vi "DistanciaRoboInimigoBola.vi"(7 "id inimigo":u32, 8 "Y bola":dbl format="%#_13g", 9 "X bola":dbl format="%#_13g", 10 "Y inimigo":dbl format="%#_13g", 11 "X inimigo":dbl format="%#_13g") -> (0 "id inimigo":u32, 3 "Distância":dbl format="%#_13g")   [LabVIEW 2017]
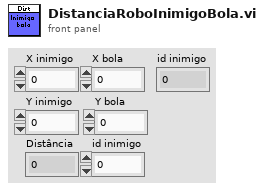
[diagram p1: front panel]
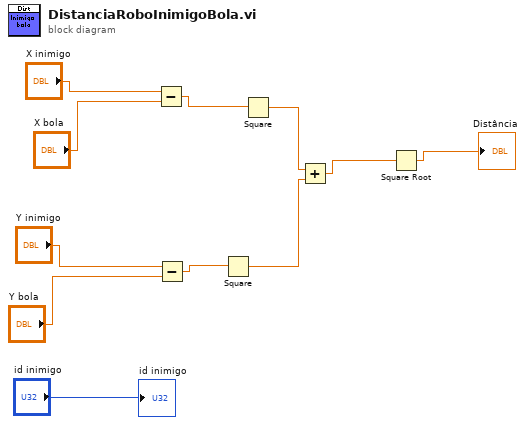
[diagram p0: block diagram]
diagram:
  n1 = Subtract(x="X inimigo", y="X bola") -> (x-y=w7:dbl)
  n2 = Subtract(x="Y inimigo", y="Y bola") -> (x-y=w6:dbl)
  n3 = Square(x=w6) -> (x^2=w4:dbl)
  n4 = Square(x=w7) -> (x^2=w5:dbl)
  n5 = Add(x=w5, y=w4) -> (x+y=w3:dbl)
  n6 = Square Root(x=w3) -> (sqrt(x)=→"Distância":dbl)
  "id inimigo" <- "id inimigo"
